vi "Get Temperature - Single.vi"(0 "reference in":refnum<class "Temp.lvclass">, 5 "error in (no error)":errorcluster) -> (14 "reference out":refnum<class "Temp.lvclass">, 16 "Temperature Channel Reading":dbl, 19 "error out":errorcluster)   [LabVIEW 2017, in "Temp.lvclass"]
uses:
  Temp.lvclass
panel:
  in  "Temperature Channel Number (Zero Based)":i32
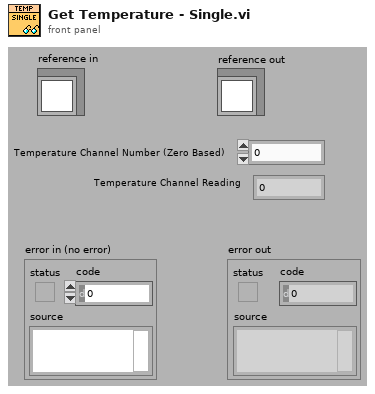
[diagram p1: front panel]
types:
  T1 = typedef "Temp.lvclass/ObjectAttributes.ctl" = cluster{"Temperature Task":refnum<k21>, "Temperature Readings":dbl[], "Thermocouple Type":i32, "Temperature Units":i32, "Average Temperature":dbl, "Number of Temperature Modules":i32, "Number of Total Temperature Channels":i32, "Temperature On/Off Status":bool, "Temperature Module Names (NI-Max Name)":string[], "Number of Channels Per Temperature  Module":i32[], "Temperature VI Reference":refnum<vi>}
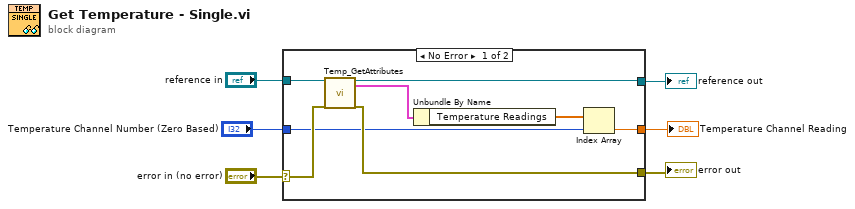
[diagram p0: block diagram]
diagram:
  n1 = case shown="No Error" "error in (no error)" {
    selector: "error in (no error)" -> [w13 w16]
    tunnel: [w11 w16] -> w5
    tunnel: [w12 w15] -> w3
    tunnel: "reference in" -> [w14 w15]
    tunnel: "Temperature Channel Number (Zero Based)" -> [w8 _]
    tunnel: [w9 _] -> w1
    frame No Error {
      n2 = call "Temp_GetAttributes.vi"("reference in"=w14, "error in (no error)"=w13) -> ("reference out"=w12:refnum<class "Temp.lvclass">, "Data"=w7:T1, "error out"=w11:errorcluster)  [unwired: 14 in, 1 out]
      n3 = Unbundle By Name(w7) -> ("Temperature Readings"=w10:dbl[])
      n4 = Index Array(array=w10, index=w8) -> (element=w9:dbl)
    }
    frame Error {
    }
  }
  "error out" <- w5
  "reference out" <- w3
  "Temperature Channel Reading" <- w1
